vi "Sort.vi"(8 "error in (no error)":errorcluster, 11 "hitRateWarning ChannelHits":refnum<vi>) -> (0 "error out":errorcluster)   [LabVIEW 2016]
uses:
  HPTDC Driver Library Folder/Library files/Typedefs/TDCHit.ctl
  Global Variables/Coincidence hunt limit.vi
  Global Variables/System info.vi
  Global Variables/Program load indicators.vi
  HPTDC Driver Library Folder/HPTDC Driver Library.lvlib
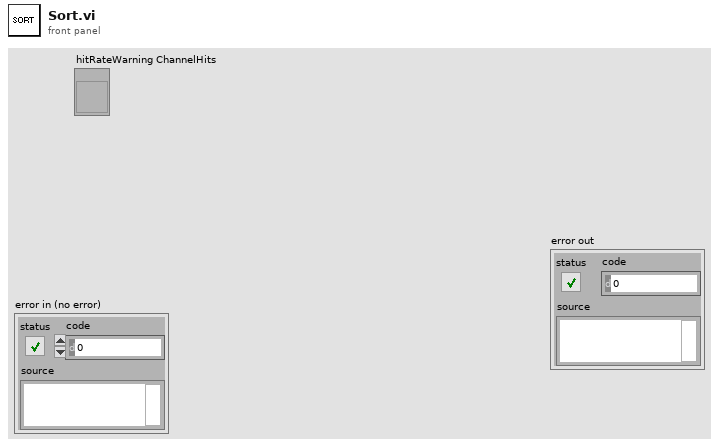
[diagram p1: front panel]
types:
  T1 = enum16{"Null", "BottomLayer", "TopAndBottom", "TopLayer"}
  T2 = typedef "HPTDC Driver Library.lvlib/TDCHit.ctl" = cluster{"channel":u8, "time":u64, "type":u8}
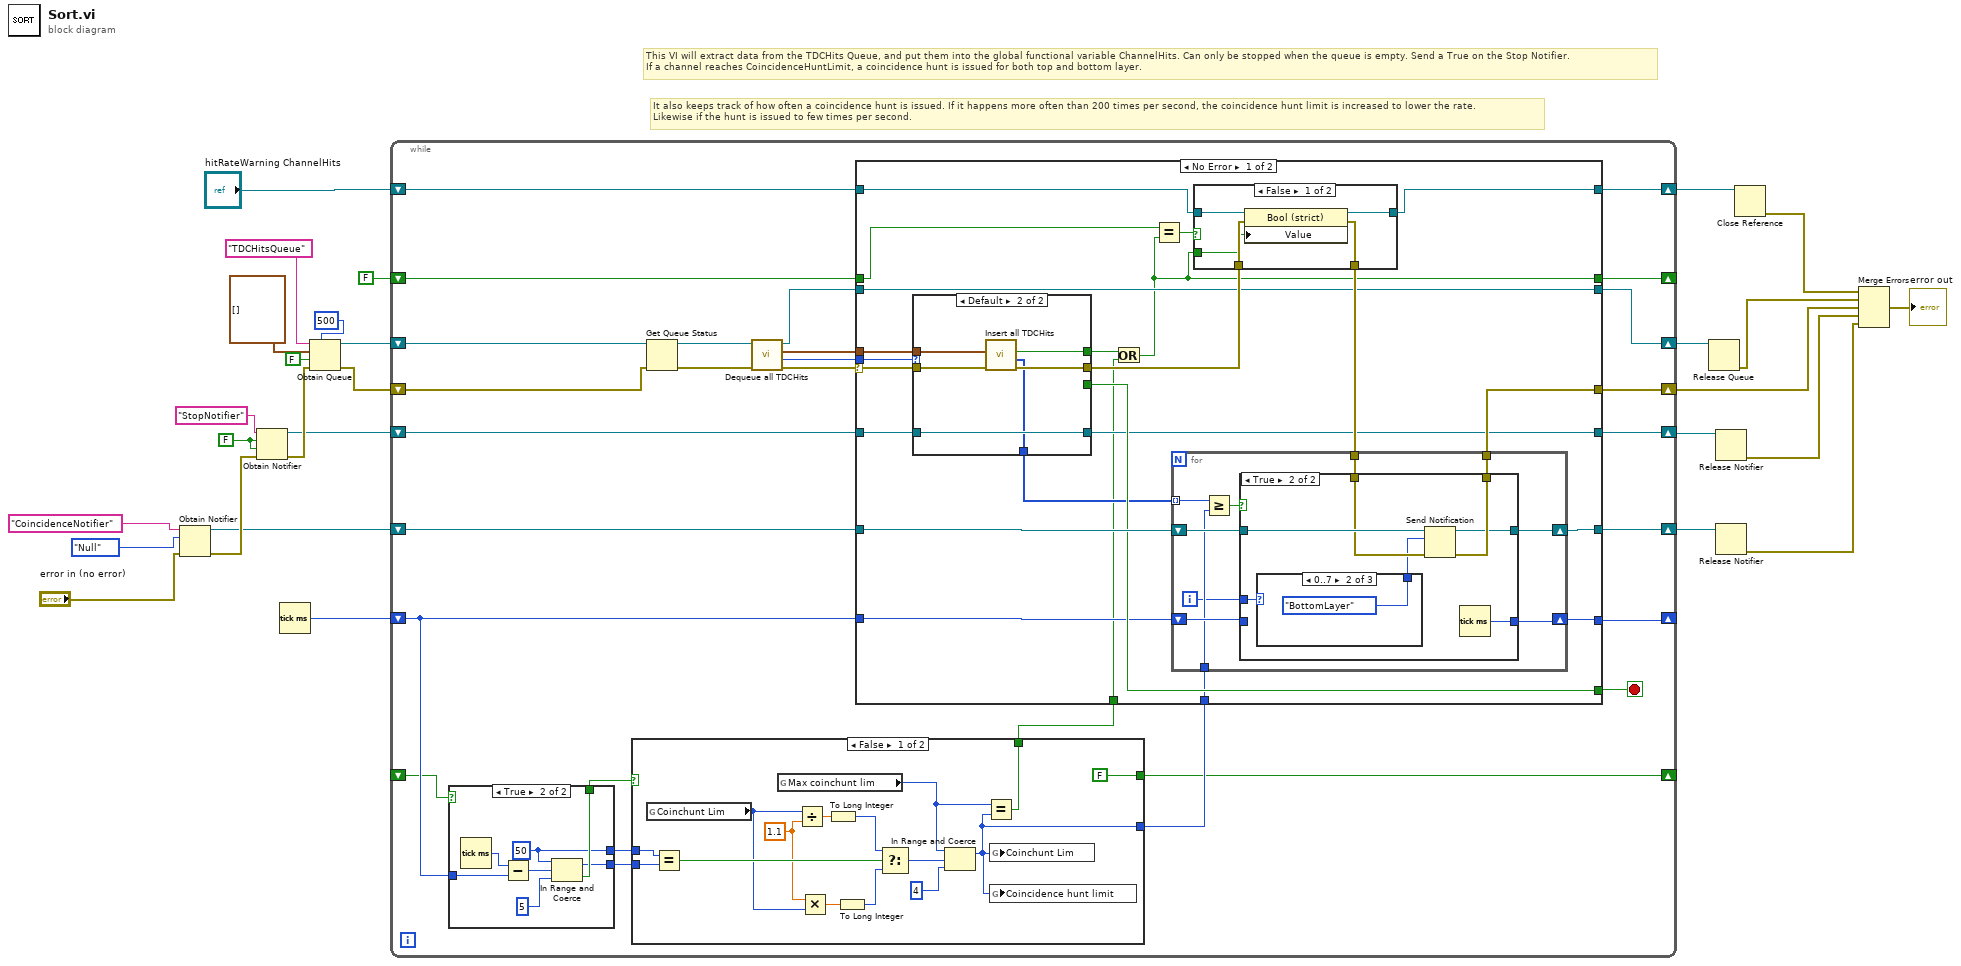
[diagram p0: block diagram]
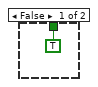
[diagram p2: hidden frame]
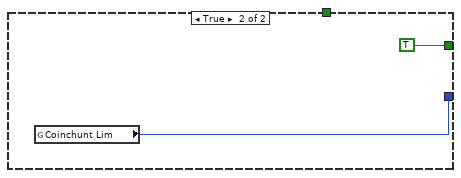
[diagram p3: hidden frame]
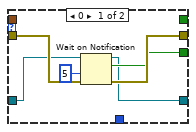
[diagram p4: hidden frame]
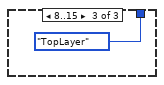
[diagram p7: hidden frame]
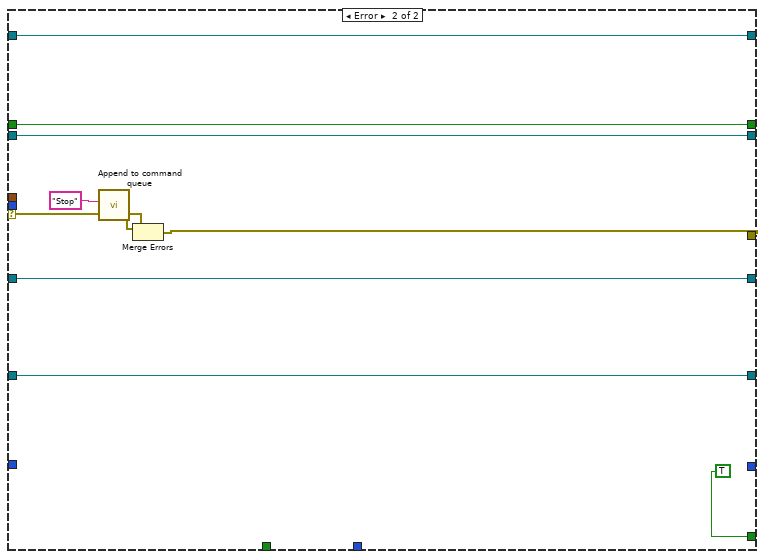
[diagram p9: hidden frame]
diagram:
  w24 = FALSE
  # "It also keeps track of how often a coincidence hunt is issued. If it happens more often than 200 times per second, the coincidence hunt limit is increased to lower the rate.\nLikewise if the hunt is issued to few times per second."
  # "This VI will extract data from the TDCHits Queue, and put them into the global functional variable ChannelHits. Can only be stopped when the queue is empty. Send a True on the Stop Notifier.\nIf a channel reaches CoincidenceHuntLimit, a coincidence hunt is issued for both top and bottom layer."
  n1 = Obtain Notifier(name (unnamed)="CoincidenceNotifier", notification data type=T1."Null" ("notification"), error in (no error)="error in (no error)") -> (notifier out=w10:refnum<notifier>, error out=w11:errorcluster)  [unwired: 1 in, 1 out]
  n2 = Obtain Notifier(name (unnamed)="StopNotifier", notification data type=w24, create if not found? (T)=w24, error in (no error)=w11) -> (notifier out=w21:refnum<notifier>, error out=w22:errorcluster)  [unwired: 1 out]
  n3 = Tick Count (ms)() -> (millisecond timer value=w2:u32)
  n4 = Obtain Queue(max queue size (-1, unlimited)=500, name (unnamed)="TDCHitsQueue", element data type=T2[] [] ("TDCHits"), create if not found? (T)=FALSE, error in (no error)=w22) -> (queue out=w3:refnum<queue>, error out=w25:errorcluster)  [unwired: 1 out]
  n5 = while {
    shift-right: [w46] -> w7
    shift-left: w25 -> [w51]
    shift-right: [w40] -> _
    shift-left: FALSE ("Buffer overflow") -> [w49]
    shift-right: [w47] -> w18
    shift-left: "hitRateWarning ChannelHits" -> [w48]
    shift-right: [w44] -> w15
    shift-left: w21 -> [w55]
    shift-right: [w43] -> w14
    shift-left: w3 -> [w53]
    shift-right: [w41] -> w9
    shift-left: w10 -> [w42]
    shift-right: [w38] -> _
    shift-left: w2 -> [w37]
    shift-right: [w32] -> _
    shift-left: _ -> [w31]
    stop <- w54 stop-if-true
    n6 = case shown="True" w31 {
      tunnel: w37 -> [_ w63]
      tunnel: [TRUE w60] -> w36
      tunnel: [_ w59] -> w35
      tunnel: [_ w58] -> w34
      frame False {
      }
      frame True {
        w58 = u32 50 ("upper limit")
        n7 = Tick Count (ms)() -> (millisecond timer value=w64:u32)
        n8 = Subtract(x=w64, y=w63) -> (x-y=w62:u32)
        n9 = In Range and Coerce(upper limit=w58, x=w62, lower limit=u32 5) -> (coerced(x)=w59:u32, In Range?=w60:bool)
      }
    }
    n10 = case shown="False" w36 {
      tunnel: w35 -> [w79 _]
      tunnel: w34 -> [w78 _]
      tunnel: [w66 w81] -> w33
      tunnel: [FALSE TRUE] -> w32
      tunnel: [w67 _] -> w30
      frame False {
        w74 = 1.1 ("y")
        n11 = global read "Coincidence hunt limit.vi" "Coinchunt Lim"() -> (w73:i32)
        n12 = Equal?(x=w78, y=w79) -> (x = y?=w76:bool)
        n13 = global read "System info.vi" "Max coinchunt lim"() -> (w65:i32)
        n14 = Divide(x=w73, y=w74) -> (x/y=w77:dbl)
        n15 = Multiply(x=w74, y=w73) -> (x*y=w69:dbl)
        n16 = To Long Integer(number=w77) -> (32bit integer=w75:i32)
        n17 = To Long Integer(number=w69) -> (32bit integer=w68:i32)
        n18 = Select(t=w75, s=w76, f=w68) -> (s? t:f=w72:i32)
        n19 = In Range and Coerce(upper limit=w65, x=w72, lower limit=4 ("upper limit")) -> (coerced(x)=w66:i32)  [unwired: 1 out]
        n20 = Equal?(x=w65, y=w66) -> (x = y?=w67:bool)
        n21 = global write "Coincidence hunt limit.vi" "Coinchunt Lim"(w66) -> ()
        n22 = global write "Program load indicators.vi" "Coincidence hunt limit"(w66) -> ()
      }
      frame True {
        n23 = global read "Coincidence hunt limit.vi" "Coinchunt Lim"() -> (w81:i32)
      }
    }
    n24 = Get Queue Status(queue=w53, error in (no error)=w51) -> (queue out=w52:refnum<queue>, error out=w50:errorcluster)  [unwired: 1 in, 6 out]
    n25 = call "Dequeue all TDCHits.vi"("error in (no error)"=w50, "Queue in"=w52) -> ("error out"=w56:errorcluster, "elements dequeued"=w39:i32, "TDCHits"=w29:T2[], "Queue out"=w45:refnum<queue>)  [unwired: 6 in]
    n26 = case shown="No Error" w56 {
      selector: w56 -> [w103 w153]
      tunnel: w29 -> [w104 _]
      tunnel: [w95 w151] -> w46
      tunnel: w55 -> [w91 w147]
      tunnel: [w90 TRUE] -> w54
      tunnel: [w83 w150] -> w40
      tunnel: w49 -> [w101 w150]
      tunnel: w48 -> [w100 w149]
      tunnel: [w99 w149] -> w47
      tunnel: w45 -> [w92 w148]
      tunnel: [w89 w147] -> w44
      tunnel: [w92 w148] -> w43
      tunnel: w42 -> [w97 w146]
      tunnel: [w94 w146] -> w41
      tunnel: w39 -> [w93 _]
      tunnel: w37 -> [w87 _]
      tunnel: [w86 _] -> w38
      tunnel: w33 -> [w85 _]
      tunnel: w30 -> [w82 _]
      frame No Error {
        n27 = case shown="Default" w93 {
          tunnel: w104 -> [_ w111]
          tunnel: w103 -> [w110 w116]
          tunnel: [w109 w115] -> w98
          tunnel: [_ w114] -> w84
          tunnel: w91 -> [w108 w113]
          tunnel: [w106 _] -> w90
          tunnel: [w105 w113] -> w89
          tunnel: [_ w112] -> w88
          frame 0 {
            n28 = Wait on Notification(notifier=w108, timeout in ms (-1)=5, error in (no error)=w110) -> (notifier out=w105:refnum<notifier>, notification=w106:bool, error out=w109:errorcluster)  [unwired: 1 in, 1 out]
          }
          frame Default {
            n29 = call "Insert all TDCHits.vi"("error in (no error)"=w116, "TDCHits"=w111) -> ("error out"=w115:errorcluster, "Nmofhits"=w112:i64[], "Buffer overflow out"=w114:bool)  [unwired: 7 in]
          }
        }
        n30 = Or(x=w84, y=w82) -> (x .or. y?=w83:bool)
        n31 = Equal?(x=w101, y=w83) -> (x = y?=w102:bool)
        n32 = case shown="False" w102 {
          tunnel: w100 -> [w143 w145]
          tunnel: w98 -> [w142 w144]
          tunnel: [w141 w144] -> w96
          tunnel: [w140 w145] -> w99
          tunnel: w83 -> [w139 _]
          frame False {
            n33 = property class="Bool (strict)"(reference=w143, error in=w142, "Value"=w139) -> (reference out=w140:refnum<vi>, error out=w141:errorcluster)
          }
          frame True {
          }
        }
        n34 = for {
          tunnel: w96 -> [w124]
          tunnel: [w123] -> w95
          shift-right: [w122] -> w94
          shift-left: w97 -> [w125]
          tunnel: w88 -> [w119] mode=indexing
          shift-right: [w118] -> w86
          shift-left: w87 -> [w121]
          tunnel: w85 -> [w120]
          i -> [w117]
          n35 = Greater Or Equal?(x=w119, y=w120) -> (x >= y?=w126:bool)
          n36 = case shown="True" w126 {
            tunnel: w125 -> [w128 w136]
            tunnel: w124 -> [w129 w135]
            tunnel: [w129 w134] -> w123
            tunnel: [w128 w133] -> w122
            tunnel: [w127 w130] -> w118
            tunnel: w121 -> [w127 _]
            tunnel: w117 -> [_ w131]
            frame False {
            }
            frame True {
              n37 = case shown="0..7" w131 {
                tunnel: [_ T1."BottomLayer" ("notification") T1."TopLayer" ("notification")] -> w132
                frame Default {
                }
                frame 0..7 {
                }
                frame 8..15 {
                }
              }
              n38 = Send Notification(notification=w132, notifier=w136, error in (no error)=w135) -> (notifier out=w133:refnum<notifier>, error out=w134:errorcluster)
              n39 = Tick Count (ms)() -> (millisecond timer value=w130:u32)
            }
          }
        }
      }
      frame Error {
        n40 = call "Append to command queue.vi"("Single command"="Stop") -> ("error out"=w152:errorcluster)  [unwired: 10 in]
        n41 = Merge Errors(w152, w153) -> (w151:errorcluster)
      }
    }
  }
  n42 = Release Queue(queue=w14) -> (error out=w8:errorcluster)  [unwired: 2 in, 2 out]
  n43 = Release Notifier(notifier=w15) -> (error out=w6:errorcluster)  [unwired: 2 in, 2 out]
  n44 = Release Notifier(notifier=w9) -> (error out=w5:errorcluster)  [unwired: 2 in, 2 out]
  n45 = Close Reference(reference=w18) -> (error out=w17:errorcluster)  [unwired: 1 in]
  n46 = Merge Errors(w17, w8, w7, w6, w5) -> (→"error out":errorcluster)
